vi "Publish Turn PID.vi"(11 "Turn By Angle":T1={"P/I/D"=[0.25, 0.001, 0.0], "Turn Speed"=0.55, "Linearity"=0.6}) -> ()   [LabVIEW 2016]
uses:
  <vilib>/Rock Robotics/Network Tables/NT Write Number.vi
  <vilib>/Rock Robotics/Network Tables/NT Write Numeric Array.vi
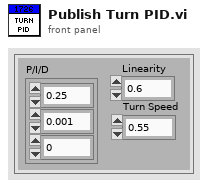
[diagram p1: front panel]
types:
  T1 = cluster{"P/I/D":dbl[], "Turn Speed":dbl, "Linearity":dbl}
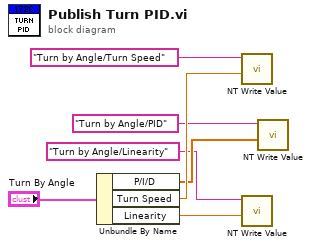
[diagram p0: block diagram]
diagram:
  n1 = Unbundle By Name("Turn By Angle") -> ("P/I/D"=w5:dbl[], "Turn Speed"=w6:dbl, "Linearity"=w7:dbl)
  n2 = call-poly <vilib>:"NT Write Value.vi"("Numeric"=w6, "Name"="Turn by Angle/Turn Speed") -> ()  [unwired: 9 in, 1 out]
  n3 = call-poly <vilib>:"NT Write Value.vi"("Numeric"=w7, "Name"="Turn by Angle/Linearity") -> ()  [unwired: 9 in, 1 out]
  n4 = call-poly <vilib>:"NT Write Value.vi"("Numeric Array"=w5, "Name"="Turn by Angle/PID") -> ()  [unwired: 9 in, 1 out]
